vi "Status Auswerten.vi"(10 "Empfangsdaten":string[](array[string])) -> (2 "Status":string, 3 "Betriebsart":string)   [LabVIEW 2020, in "Linearisierung v2.lvlib" / "Gasteiler.lvlib" / "AK Komm Gasteiler.lvlib"]
uses:
  AK Komm Gasteiler.lvlib
  Aktionen FGV Gasteiler Daten.ctl
  Gasteiler.lvlib
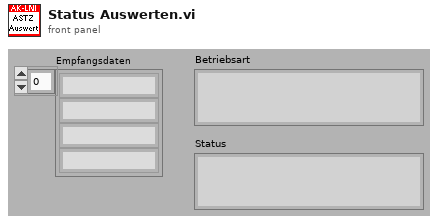
[diagram p1: front panel]
types:
  T1 = typedef "Linearisierung v2.lvlib/Gasteiler.lvlib/Aktionen FGV Gasteiler Daten.ctl" = enum16{"lesen", "Gasteiler Daten", "Seriellen Param.", "MB-Endwert", "laden", "speichern", "Anforderung", "TCP", "Aufzeichnung Start"}
  T2 = typedef "Linearisierung v2.lvlib/GasteilerType.ctl" = u16
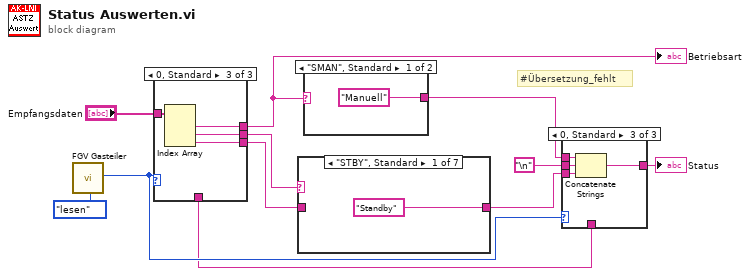
[diagram p0: block diagram]
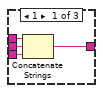
[diagram p2: hidden frame]
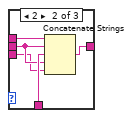
[diagram p3: hidden frame]
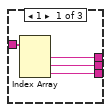
[diagram p4: hidden frame]
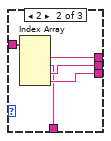
[diagram p5: hidden frame]
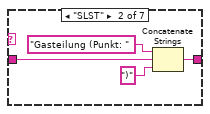
[diagram p6: hidden frame]
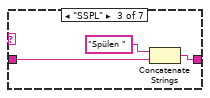
[diagram p7: hidden frame]
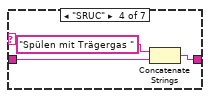
[diagram p8: hidden frame]
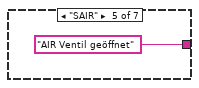
[diagram p9: hidden frame]
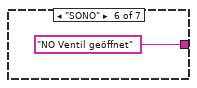
[diagram p10: hidden frame]
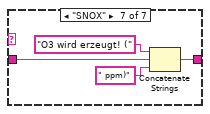
[diagram p11: hidden frame]
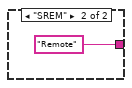
[diagram p12: hidden frame]
diagram:
  # "#Übersetzung_fehlt"
  n1 = call "FGV Gasteiler.vi"("Aktionen"=Aktionen_FGV_Gasteiler_Daten."lesen") -> ("Gasteiler Type"=w3:T2)  [unwired: 11 in, 7 out]
  n2 = case shown="0, Standard" w3 {
    tunnel: "Empfangsdaten" -> [w15 w20 w24]
    tunnel: [w14 w19 w23] -> w1
    tunnel: [w13 w18 w22] -> w10
    tunnel: [w12 w17 w21] -> w9
    tunnel: [_ w16 _] -> w2
    frame 1 {
      n3 = Index Array(array=w15) -> (element #1=w14:string, element #2=w13:string, element #3=w12:string)  [unwired: 3 in]
    }
    frame 2 {
      n4 = Index Array(array=w20) -> (element #1=w19:string, element #2=w16:string, element #3=w18:string, element #4=w17:string)  [unwired: 4 in]
    }
    frame 0, Default {
      n5 = Index Array(array=w24) -> (element #1=w23:string, element #2=w22:string, element #3=w21:string)  [unwired: 3 in]
    }
  }
  "Betriebsart" <- w1
  n6 = case shown="\"STBY\", Standard" w10 {
    tunnel: w9 -> [_ w28 w31 w34 _ _ w40]
    tunnel: ["Standby" w26 w30 w33 "AIR Ventil geöffnet" "NO Ventil geöffnet" w39] -> w6
    frame "STBY", Default {
    }
    frame "SLST" {
      n7 = Concatenate Strings("Gasteilung (Punkt: ", w28, ")" ("String")) -> (w26:string)
    }
    frame "SSPL" {
      n8 = Concatenate Strings("Spülen ", w31) -> (w30:string)
    }
    frame "SRUC" {
      n9 = Concatenate Strings("Spülen mit Trägergas ", w34) -> (w33:string)
    }
    frame "SAIR" {
    }
    frame "SONO" {
    }
    frame "SNOX" {
      n10 = Concatenate Strings("O3 wird erzeugt! (", w40, " ppm)" ("String")) -> (w39:string)
    }
  }
  n11 = case shown="\"SMAN\", Standard" w1 {
    tunnel: ["Manuell" "Remote"] -> w8
    frame "SMAN", Default {
    }
    frame "SREM" {
    }
  }
  n12 = case shown="0, Standard" w3 {
    tunnel: w8 -> [w47 w52 w56]
    tunnel: "\n" -> [w46 w49 w55]
    tunnel: w6 -> [w45 w48 w54]
    tunnel: [w44 w51 w53] -> w5
    tunnel: w2 -> [_ w50 _]
    frame 1 {
      n13 = Concatenate Strings(w47, w46, w45) -> (w44:string)
    }
    frame 2 {
      n14 = Concatenate Strings(w52, w49, w50, w49, w48) -> (w51:string)
    }
    frame 0, Default {
      n15 = Concatenate Strings(w56, w55, w54) -> (w53:string)
    }
  }
  "Status" <- w5
